vi "streaming.vi"() -> ()   [LabVIEW 2012]
uses:
  wlcomp.dll
panel:
  out "error out":errorcluster
  in  "error in (no error)":errorcluster
  in  "Offset_I":dbl=77.0
  in  "Coeff_I":dbl=42.391
  in  "Offset_U":dbl=6.5
  in  "Coeff_U":dbl=2.55
  out "Time_indicator":dbl format="%.1f"
  out "Ik''amp":dbl format="%.2f"
  out "IK''ef":dbl format="%.2f"
  out "Ik''av":dbl format="%.2f"
  out "Ia''amp":dbl format="%.2f"
  out "Ia''ef":dbl format="%.2f"
  out "Ia''av":dbl format="%.2f"
  out "Uk''amp":dbl format="%.1f"
  out "Uk''ef":dbl format="%.1f"
  out "Uk''av":dbl format="%.1f"
  out "Ua''amp":dbl format="%.1f"
  out "Ua''ef":dbl format="%.1f"
  out "Ua''av":dbl format="%.1f"
  out "Ток":dbl[](graph)
  out "Напряжение":dbl[](graph)
  in  "Стоп":bool
  out "BoardType":u32
  out "Dsp":u32
  out "Irq":u32
  out "Base I/O":u32 format="%.0x"
  out "SerNum":string
  out "BrdName":string
  out "Rev":string
  out "DspType":string
  out "Quartz":i32
  out "IsDacPresent":u16
  out "Error":u32
  out "Alloc":u32
  out "IrqStep":u32
  out "FIFO":u32
  out "dRate":dbl format="%.2f"
  out "Pages":u32
  out "size":u32
  out "sync addr":u32
  out "data addr":u32
  out "sync counter":u32
  in  "Enter bios name":string="l761"
  in  "Enter slot number":u32
  out "TTL Input (IoAsync demo)":i32
  out "Numeric":i32
  # "Напряжение"
  # "Ток"
  # "Анодное"
  # "Катодное"
  # "Анодный"
  # "Катодный"
  # "Среднее"
  # "Действующее"
  # "Амплитудное"
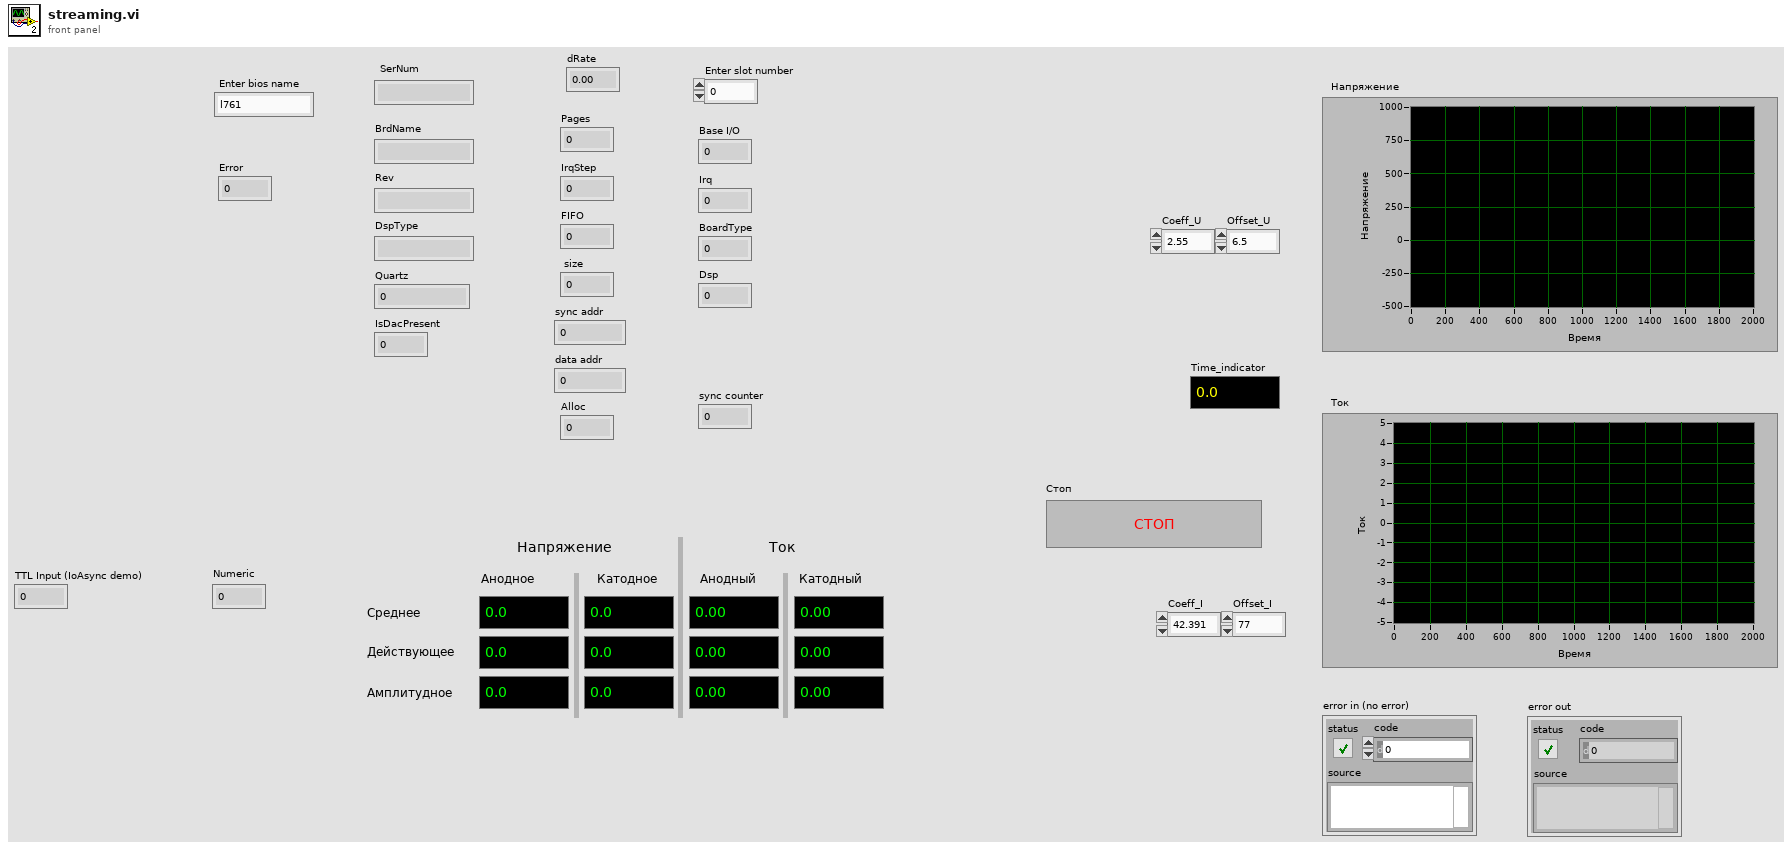
[diagram p1: front panel]
types:
  T1 = cluster{"s_Type":u32, "FIFO":u32, "IrqStep":u32, "Pages":u32, "Autoinit":u32, "dRate":dbl, "dKadr":dbl, "dScale":dbl, "Rate":u32, "Kadr":u32, "Scale":u32, "FPDelay":u32, "SynchroType\n3 - without sync(L7XX E2010)\n0 - without sync(E440 E140 E154 L791)":u32, "SynchroSensitivity":u32, "SynchroMode":u32, "AdChannel":u32, "AdPorog":u32, "NCh":u32, u32[], "IrqEna":u32, "AdcEna":u32}
  T2 = cluster{"[0]":u32, "[1]":u32, "[2]":u32, "[3]":u32, "[4]":u32, "[5]":u32, "[6]":u32, "[7]":u32, "[8]":u32, "[9]":u32, "[10]":u32, "[11]":u32, "[12]":u32, "[13]":u32, "[14]":u32, "[15]":u32, "[16]":u32, "[17]":u32, "[18]":u32, "[19]":u32}
  T3 = cluster{string, string, string, string, i32, u16}
  T4 = cluster{"s_Type":u32, "FIFO":u32, "IrqStep":u32, "Pages":u32, "dRate":dbl, "Rate":u32, "NCh":u32, "Chn[0]":u32, "Data[0]":u32, "Mode":u32}
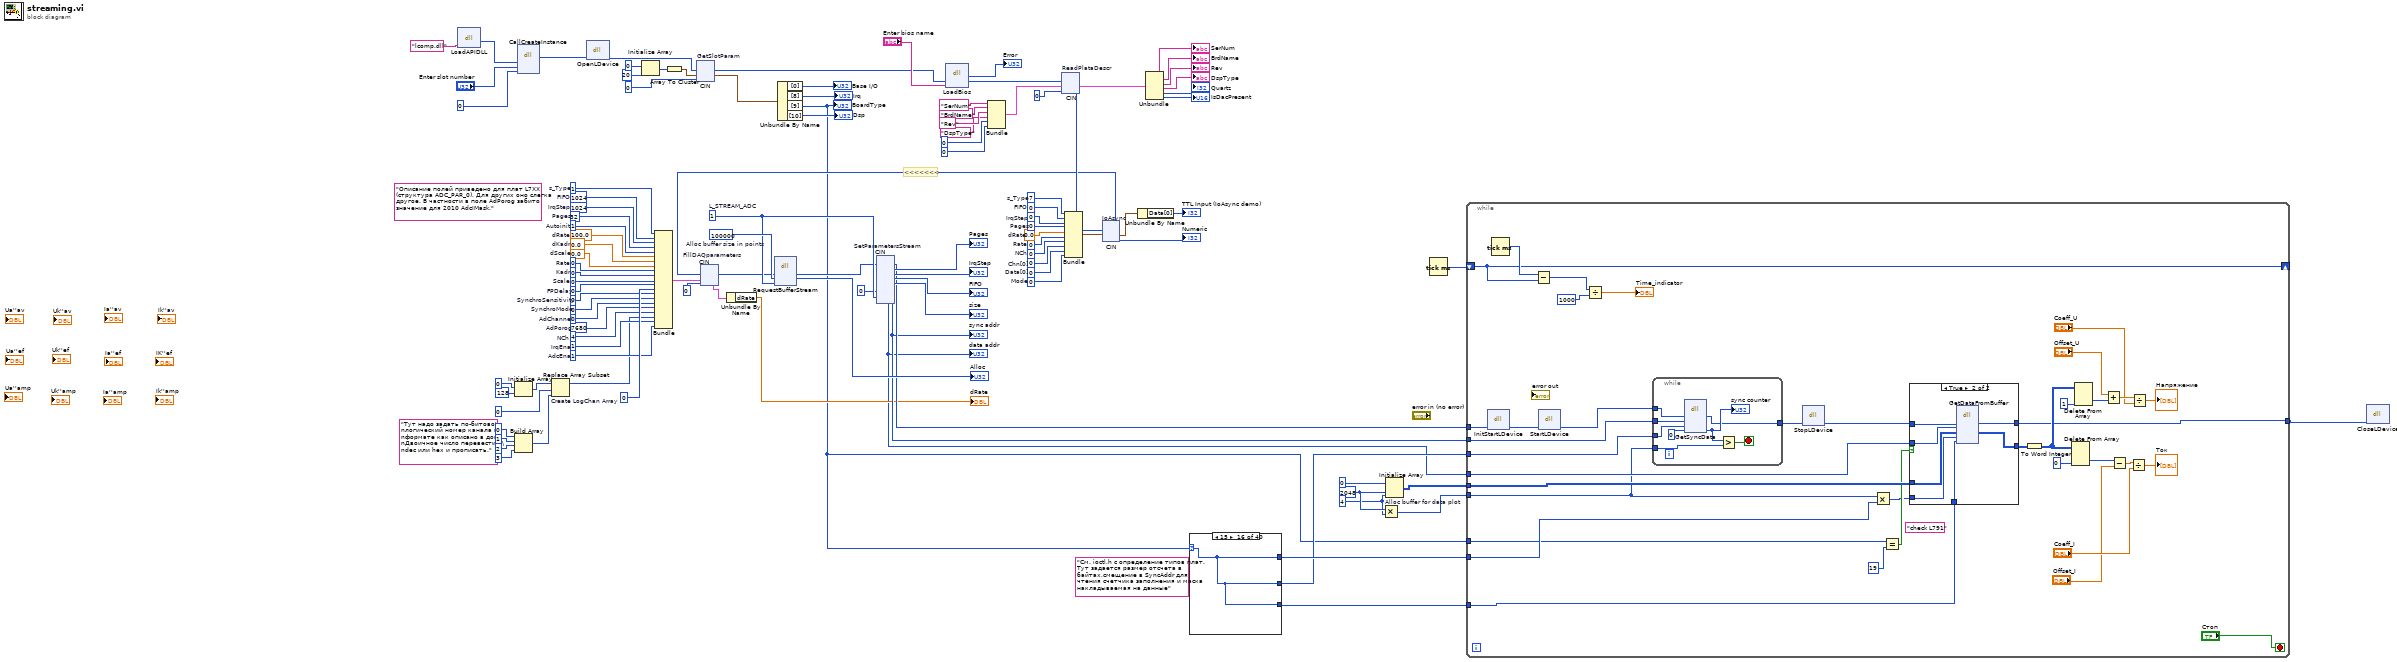
[diagram p0: block diagram]
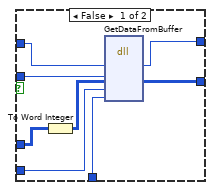
[diagram p2: hidden frame]
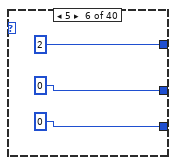
[diagram p8: hidden frame]
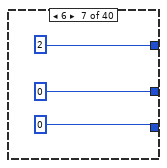
[diagram p9: hidden frame]
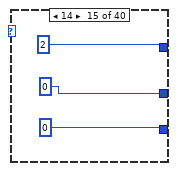
[diagram p17: hidden frame]
diagram:
  (unwired) "Тут надо задать по-битово\nлогический номер канала в \nформате как описано в док.\nДвоичное число перевести в\ndec или hex и прописать."
  (unwired) "См. ioctl.h с определение типов плат. Тут задается размер отсчета в байтах,смещение в SyncAddr для чтения счетчика заполнения и маска накладываемая на данные"
  (unwired) "Описание полей приведено для плат L7XX (структура ADC_PAR_0). Для других оно слегка другое. В частности в поле AdPorog забито значение для 2010 AdcIMask."
  w28 = u32 0  # Mode
  w19 = u32 0  # Data[0]
  w20 = u32 0  # Chn[0]
  w21 = u32 0  # NCh
  w22 = u32 0  # Rate
  w23 = 0.0  # dRate
  w24 = u32 0  # Pages
  w25 = u32 0  # IrqStep
  w26 = u32 0  # FIFO
  w27 = u32 7  # s_Type
  w29 = 4
  w48 = 2048
  w54 = u32 1  # L_STREAM_ADC
  w55 = u32 100000  # Alloc buffer size in points
  w66 = u32 1  # AdcEna
  w67 = u32 1  # IrqEna
  w68 = u32 4  # NCh
  w69 = u32 7680  # AdPorog
  w70 = u32 0  # AdChannel
  w71 = u32 0  # SynchroMode
  w72 = u32 0  # SynchroSensitivity
  w74 = u32 0  # FPDelay
  w75 = u32 0  # Scale
  w76 = u32 0  # Kadr
  w77 = u32 0  # Rate
  w78 = 0.0  # dScale
  w79 = 0.0  # dKadr
  w80 = 100.0  # dRate
  w81 = u32 1  # Autoinit
  w82 = u32 32  # Pages
  w83 = u32 1024  # IrqStep
  w84 = u32 1024  # FIFO
  w85 = u32 1  # s_Type
  # "<<<<<<<"
  n1 = dll-call lib="wlcomp.dll" fn="LoadAPIDLL" label="LoadAPIDll"("dllname"="lcomp.dll") -> (w107:u32)  [unwired: 4 in, 2 out]
  n2 = Initialize Array(u32 0, u32 128) -> (w63:u32[])
  n3 = Build Array(0, 1, 2, 3) -> (w60:i32[])
  n4 = dll-call lib="wlcomp.dll" fn="CallCreateInstance"("hDll"=w107, "slot"="Enter slot number", "Err"=u32 0) -> (w44:u32)  [unwired: 6 in, 2 out]
  n5 = Replace Array Subset "Create LogChan Array"(array=w63, new element=w60, index=u32 0) -> (w62:u32[])
  n6 = dll-call lib="wlcomp.dll" fn="OpenLDevice"("hIfc"=w44) -> ("hIfc"=w43:u32)  [unwired: 4 in, 2 out]
  n7 = Initialize Array(u32 0, u32 20) -> (w104:u32[])
  n8 = Bundle("s_Type"=w85, "FIFO"=w84, "IrqStep"=w83, "Pages"=w82, "Autoinit"=w81, "dRate"=w80, "dKadr"=w79, "dScale"=w78, "Rate"=w77, "Kadr"=w76, "Scale"=w75, "FPDelay"=w74, "SynchroType\n3 - without sync(L7XX E2010)\n0 - without sync(E440 E140 E154 L791)"=u32 0 ("SynchroType\n3 - without sync(L7XX E2010)\n0 - without sync(E440 E140 E154 L791)"), "SynchroSensitivity"=w72, "SynchroMode"=w71, "AdChannel"=w70, "AdPorog"=w69, "NCh"=w68, w62, "IrqEna"=w67, "AdcEna"=w66) -> (w86:T1)  [unwired: 1 in]
  n9 = Array To Cluster(array=w104) -> (cluster=w100:T2)
  n10 = cin "GetSlotParam"(w43, w100, u32 0) -> (w37:u32, w11:T2)  [unwired: 1 in]
  n11 = Unbundle By Name(w11) -> ("[0]"=→"Base I/O":u32, "[8]"=→"Irq":u32, "[9]"=w5:u32, "[10]"=→"Dsp":u32)
  "BoardType" <- w5
  n12 = dll-call lib="wlcomp.dll" fn="LoadBios"("hIfc"=w37, "BiosName"="Enter bios name") -> (→"Error":u32, "hIfc"=w36:u32)  [unwired: 4 in, 2 out]
  n13 = Bundle("SerNum", "BrdName", "Rev", "DspType", 0, u16 0) -> (w33:T3)  [unwired: 1 in]
  n14 = cin "ReadPlataDescr"(w36, w33, u32 0) -> (w15:u32, w93:T3)  [unwired: 1 in]
  n15 = Bundle("s_Type"=w27, "FIFO"=w26, "IrqStep"=w25, "Pages"=w24, "dRate"=w23, "Rate"=w22, "NCh"=w21, "Chn[0]"=w20, "Data[0]"=w19, "Mode"=w28) -> (w18:T4)  [unwired: 1 in]
  n16 = cin "IoAsync"(w15, w18) -> (w13:u32, w4:T4, →"Numeric":i32)  [unwired: 1 in]
  n17 = cin "FillDAQparameters"(w13, w86, 0) -> (w40:u32, w7:T1)  [unwired: 1 in]
  n18 = Unbundle By Name(w7) -> ("dRate"=→"dRate":dbl)
  n19 = dll-call lib="wlcomp.dll" fn="RequestBufferStream" label="RequestBuffer"("hIfc"=w40, "Size"=w55, "StreamId"=w54) -> ("hIfc"=w39:u32, "Size"=→"Alloc":u32)  [unwired: 5 in, 2 out]
  n20 = cin "SetParametersStream"(w39, w54, u32 0) -> (w14:u32, →"Pages":u32, →"IrqStep":u32, →"FIFO":u32, →"size":u32, w12:u32, w1:u32)  [unwired: 8 in]
  "sync addr" <- w12
  "data addr" <- w1
  n21 = Unbundle By Name(w4) -> ("Data[0]"=→"TTL Input (IoAsync demo)":u32)
  n22 = Unbundle(w93) -> (→"SerNum":string, →"BrdName":string, →"Rev":string, →"DspType":string, →"Quartz":i32, →"IsDacPresent":u16)
  n23 = case shown="15" w5 {
    selector: w5 -> [w109 w110 w111 w112 w113 _ _ w120 w121 w122 w123 w124 w125 w126 _ w130 w131 w132 w133 _ w137 w138 w139 w140 w141 w142 w143 w144 w145 w146 _ _ _ w156 w157 w158 w159 w160 _ _]
    tunnel: [w109 w110 w111 w112 w113 2 2 w120 w121 w122 w123 w124 w125 w126 2 w130 w131 w132 w133 4 w137 w138 w139 w140 w141 w142 w143 w144 w145 w146 2 2 2 w156 w157 w158 w159 w160 2 2] -> w32
    tunnel: [w109 w110 w111 w112 w113 0 0 w120 w121 w122 w123 w124 w125 w126 0 w130 w131 w132 w133 992 w137 w138 w139 w140 w141 w142 w143 w144 w145 w146 0 0 0 w156 w157 w158 w159 w160 0 0] -> w31
    tunnel: [w109 w110 w111 w112 w113 0 0 w120 w121 w122 w123 w124 w125 w126 0 w130 w131 w132 w133 65535 w137 w138 w139 w140 w141 w142 w143 w144 w145 w146 0 0 0 w156 w157 w158 w159 w160 0 0] -> w30
    frame 0, Default {
    }
    frame 1 {
    }
    frame 2 {
    }
    frame 3 {
    }
    frame 4 {
    }
    frame 5 {
    }
    frame 6 {
    }
    frame 7 {
    }
    frame 8 {
    }
    frame 9 {
    }
    frame 10 {
    }
    frame 11 {
    }
    frame 12 {
    }
    frame 13 {
    }
    frame 14 {
    }
    frame 15 {
    }
    frame 16 {
    }
    frame 17 {
    }
    frame 18 {
    }
    frame 19 {
    }
    frame 20 {
    }
    frame 21 {
    }
    frame 22 {
    }
    frame 23 {
    }
    frame 24 {
    }
    frame 25 {
    }
    frame 26 {
    }
    frame 27 {
    }
    frame 28 {
    }
    frame 29 {
    }
    frame 30 {
    }
    frame 31 {
    }
    frame 32 {
    }
    frame 33 {
    }
    frame 34 {
    }
    frame 35 {
    }
    frame 36 {
    }
    frame 37 {
    }
    frame 38 {
    }
    frame 39 {
    }
  }
  n24 = Multiply(x=w48, y=w29) -> (x*y=w46:i32)
  n25 = Initialize Array "Alloc buffer for data plot"(u32 0, w48, w29) -> (w47:u32[][])
  n26 = Tick Count (ms)() -> (millisecond timer value=w2:u32)
  n27 = while {
    tunnel: w47 -> [w203]
    tunnel: w46 -> [w187]
    tunnel: [w171] -> w45
    tunnel: w32 -> [w202]
    tunnel: w31 -> [w188]
    tunnel: w30 -> [w201]
    tunnel: w14 -> [w192]
    tunnel: w5 -> [w200]
    tunnel: w12 -> [w189]
    shift-right: [w196] -> _
    shift-left: w2 -> [w196]
    tunnel: w1 -> [w191]
    stop <- "Стоп" stop-if-true
    (unwired) "check L791"
    n28 = dll-call lib="wlcomp.dll" fn="InitStartLDevice"("hIfc"=w192) -> ("hIfc"=w193:u32)  [unwired: 4 in, 2 out]
    n29 = Tick Count (ms)() -> (millisecond timer value=w199:u32)
    n30 = Subtract(x=w199, y=w196) -> (x-y=w198:u32)
    n31 = dll-call lib="wlcomp.dll" fn="StartLDevice"("hIfc"=w193) -> ("hIfc"=w190:u32)  [unwired: 4 in, 2 out]
    n32 = Divide(x=w198, y=1000) -> (x/y=→"Time_indicator":dbl)
    n33 = while {
      tunnel: w190 -> [w226]
      tunnel: w188 -> [w223]
      tunnel: w187 -> [w221]
      tunnel: w189 -> [w220]
      tunnel: [w219] -> w186
      stop <- w222 stop-if-true
      n34 = dll-call lib="wlcomp.dll" fn="GetSyncData"("hIfc"=w226, "sync"=w220, "offs"=w223, "sincd"=u32 0) -> ("hIfc"=w219:u32, "sincd"=w225:u32)  [unwired: 6 in, 2 out]
      "sync counter" <- w225
      n35 = Greater?(x=w225, y=w221) -> (0:w222:bool)
    }
    n36 = dll-call lib="wlcomp.dll" fn="StopLDevice"("hIfc"=w186) -> ("hIfc"=w172:u32)  [unwired: 4 in, 2 out]
    n37 = Multiply(x=w187, y=w202) -> (x*y=w183:u32)
    n38 = Equal?(x=w200, y=19) -> (x = y?=w184:bool)
    n39 = case shown="True" w184 {
      tunnel: w172 -> [w211 w218]
      tunnel: w191 -> [w210 w217]
      tunnel: w203 -> [w207 w216]
      tunnel: w183 -> [w209 w215]
      tunnel: w201 -> [w208 w214]
      tunnel: [w205 w213] -> w173
      tunnel: [w204 w212] -> w171
      frame False {
        n40 = To Word Integer(number=w207) -> (16bit integer=w206:i16[][])
        n41 = dll-call lib="wlcomp.dll" fn="GetDataFromBuffer"("hIfc"=w211, "data"=w210, "datad"=w206, "size"=w209, "mask"=w208) -> ("hIfc"=w204:u32, "datad"=w205:i16[][])  [unwired: 7 in, 2 out]
      }
      frame True {
        n42 = dll-call lib="wlcomp.dll" fn="GetDataFromBuffer"("hIfc"=w218, "data"=w217, "datad"=w216, "size"=w215, "mask"=w214) -> ("hIfc"=w212:u32, "datad"=w213:u32[][])  [unwired: 7 in, 2 out]
      }
    }
    n43 = To Word Integer(number=w173) -> (16bit integer=w181:i16[][])
    n44 = Delete From Array(array=w181, index (col)=0 ("disabled index (col)")) -> (deleted portion=w177:i16[])  [unwired: 2 in, 1 out]
    n45 = Delete From Array(array=w181, index (col)=1 ("disabled index (col)")) -> (deleted portion=w179:i16[])  [unwired: 2 in, 1 out]
    n46 = Add(x="Offset_U", y=w179) -> (x+y=w178:dbl[])
    n47 = Subtract(x=w177, y="Offset_I") -> (x-y=w176:dbl[])
    n48 = Divide(x=w176, y="Coeff_I") -> (x/y=→"Ток":dbl[])
    n49 = Divide(x=w178, y="Coeff_U") -> (x/y=→"Напряжение":dbl[])
  }
  n50 = dll-call lib="wlcomp.dll" fn="CloseLDevice"("hIfc"=w45) -> ()  [unwired: 5 in, 2 out]
